vi "Remove Tree Underscore.vi"(0 "Input String":string="Demosa_2") -> (1 "Data":string, 2 "Removed":string)   [LabVIEW 2020]
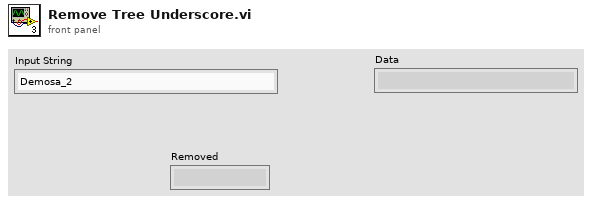
[diagram p1: front panel]
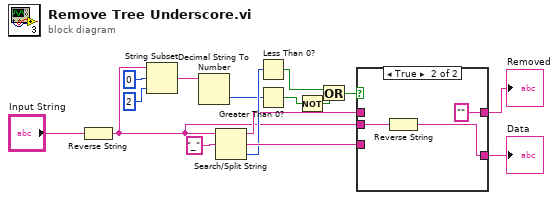
[diagram p0: block diagram]
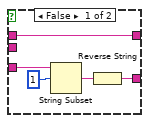
[diagram p2: hidden frame]
diagram:
  n1 = Reverse String(1:"Input String") -> (0:w9:string)
  n2 = String Subset(string=w9, offset (0)=0, length (rest)=2 ("length (rest)")) -> (substring=w6:string)
  n3 = Decimal String To Number(string=w6) -> (number=w3:i32)  [unwired: 2 in, 1 out]
  n4 = Search/Split String(string=w9, search string/char (-)="_") -> (substring before match=w10:string, match + rest of string=w14:string, offset of match=w12:i32)  [unwired: 1 in]
  n5 = Less Than 0?(x=w12) -> (x < 0?=w4:bool)
  n6 = Greater Than 0?(x=w3) -> (x > 0?=w1:bool)
  n7 = Not(x=w1) -> (.not. x?=w2:bool)
  n8 = Or(x=w4, y=w2) -> (x .or. y?=w5:bool)
  n9 = case shown="True" w5 {
    tunnel: w14 -> [w21 _]
    tunnel: [w18 w23] -> w13
    tunnel: w9 -> [_ w24]
    tunnel: [w17 "" ("Removed")] -> w11
    tunnel: w10 -> [w17 _]
    frame False {
      n10 = String Subset(string=w21, offset (0)=1) -> (substring=w19:string)  [unwired: 1 in]
      n11 = Reverse String(1:w19) -> (0:w18:string)
    }
    frame True {
      n12 = Reverse String(1:w24) -> (0:w23:string)
    }
  }
  "Removed" <- w11
  "Data" <- w13
